vi "Append Image to Report (path).vi"(0 "report in":refnum<class "NI_Standard Report.lvclass">, 1 "alignment (default)":T1, 2 "MS Office parameters":T2, 7 "path or URL of image":path, 9 "caption or alternative string":string, 11 "error in (no error)":errorcluster) -> (4 "report out":refnum<class "NI_Standard Report.lvclass">, 8 "start out (Word)":i32, 10 "end out (Word)":i32, 15 "error out":errorcluster)   [LabVIEW 2015, in "NI_Standard Report.lvclass"]
doc: "For an HTML report, the VI embeds a link to an image into the report. For a standard report, the VI appends the image from a file. You can wire either a path to the image or a string that contains the image URL to this polymorphic VI. The data type you wire to the <B>path or URL of image</B> input determines the polymorphic instance to use."
uses:
  <vilib>/Utility/NIReport.llb/Standard Report/NI_Standard Report.lvclass
  <vilib>/Utility/NIReport.llb/HTML Report Image Alignment.ctl
  <vilib>/Utility/NIReport.llb/Standard Report/NI_Standard Report.lvclass/NI_Standard Report.ctl
  <vilib>/Utility/NIReport.llb/NI_ReportGenerationCore.lvlib
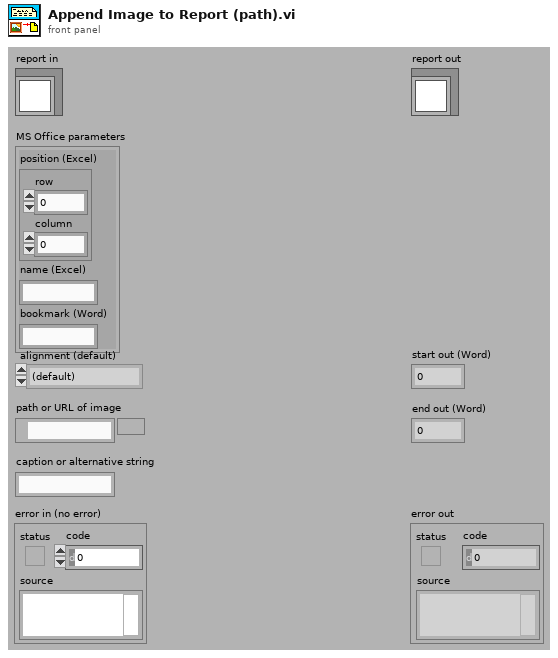
[diagram p1: front panel]
types:
  T1 = typedef "NI_ReportGenerationCore.lvlib/HTML Report Image Alignment.ctl" = enum16{"(default)", "LEFT", "RIGHT", "TOP", "TEXTTOP", "MIDDLE", "ABSMIDDLE", "BASELINE", "BOTTOM", "ABSBOTTOM"}
  T2 = cluster{"position (Excel)":cluster{"row":i32, "column":i32}, "name (Excel)":string, "bookmark (Word)":string}
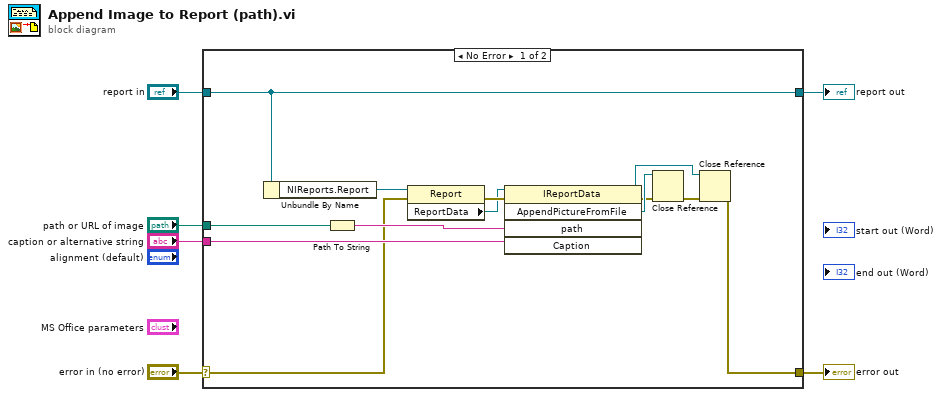
[diagram p0: block diagram]
diagram:
  n1 = case shown="No Error" "error in (no error)" {
    selector: "error in (no error)" -> [w9 w21]
    tunnel: [w8 w21] -> w5
    tunnel: [w7 w20] -> w3
    tunnel: "report in" -> [w7 w20]
    tunnel: "path or URL of image" -> [w11 _]
    tunnel: "caption or alternative string" -> [w10 _]
    frame No Error {
      n2 = Unbundle By Name(w7) -> ("NIReports.Report"=w12:refnum<k7>)
      n3 = Path To String(path=w11) -> (string=w13:string)
      n4 = property class="Report"(reference=w12, error in=w9) -> (error out=w15:errorcluster, "ReportData"=w14:refnum<k7>)  [unwired: 1 out]
      n5 = invoke class="IReportData" method="AppendPictureFromFile"(reference=w14, error in=w15, "path"=w13, "Caption"=w10) -> (reference out=w19:refnum<k7>, error out=w17:errorcluster, "AppendPictureFromFile"=w18:refnum<k7>)  [unwired: 1 in, 2 out]
      n6 = Close Reference(reference=w18, error in (no error)=w17) -> (error out=w16:errorcluster)
      n7 = Close Reference(reference=w19, error in (no error)=w16) -> (error out=w8:errorcluster)
    }
    frame Error {
    }
  }
  "error out" <- w5
  "report out" <- w3
